vi "Plot Name Write.vi"(4 "error in (no error)":errorcluster, 5 "Value":string, 6 "Container State":T3, 7 "Display State In":T1) -> (0 "error out":errorcluster, 3 "Display State Out":T1)   [LabVIEW 2020, in "XY Plot Matrix.xctl"]
uses:
  <vilib>/Math Plots/2D Math Plots/XY Plot Matrix/XY Plot Matrix XCtrl/XY Plot Matrix.xctl
  <vilib>/_xctls/Container State.ctl
  <vilib>/Math Plots/2D Math Plots/XY Plot Matrix/XY Plot Matrix XCtrl/State.ctl
  <vilib>/Math Plots/2D Math Plots/XY Plot Matrix/XY Plot Matrix/XY Plot Matrix.lvclass
  e:/builds/penguin/labview/branches/2020/dev/dist/vi.lib/Math Plots/2D Math Plots/2D Plot/2D Plot/2D Plot.lvclass
  <vilib>/Math Plots/2D Math Plots/2D Plot/Action String/XYPlotMatrix Ctrl Act Queue.ctl
  <vilib>/Math Plots/2D Math Plots/2D Plot/Action String/XYPlotMatrix Ctrl Act Cluster.ctl
  <vilib>/Math Plots/2D Math Plots/2D Plot/Action String/2DMathPlot State Class.ctl
  <vilib>/Math Plots/2D Math Plots/2D Plot/2D Plot/2D Plot.lvclass
  <vilib>/_xctls/XControlSupport.lvlib
panel:
  # "Replace the Value Control below with a Control of desired type.\nDo not remove this Control or the others from the connector pane.\nDo not change the connector pane pattern.\nThe Value control should always be the third terminal from top on the input side in the connector pane."
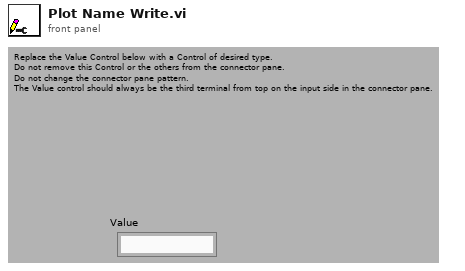
[diagram p1: front panel]
types:
  T1 = typedef "XY Plot Matrix.xctl/State.ctl" = cluster{"XY Plot Matrix.lvclass":refnum<class "XY Plot Matrix.lvclass">, "Control Ref Queue":T2, "Main Frame Color":u32}
  T2 = typedef "XYPlotMatrix Ctrl Act Queue.ctl" = refnum<queue>
  T3 = typedef "XControlSupport.lvlib/Container State.ctl" = cluster{"Indicator?":bool, "Run Mode?":bool, " Refnum":refnum<vi>}
  T4 = typedef "2DMathPlot State Class.ctl" = enum16{"Update All (Undo)", "Update General", "Update Appearance", "Update Format", "Update Scale", "Update Marker", "Update Cursor", "None"}
  T5 = typedef "XY Plot Matrix.lvclass/Plotmatrix Property Array Cluster.ctl" = cluster{"Plotmatrix Property Array":T6, "Active Position":T10}
  T6 = typedef "XY Plot Matrix.lvclass/Plotmatrix Property Array.ctl" = T7[][]
  T7 = typedef "XY Plot Matrix.lvclass/Plotmatrix Property.ctl" = cluster{"Plot Property Array":T8}
  T8 = typedef "2D Plot.lvclass/Plot Property Array.ctl" = T9[]
  T9 = typedef "2D Plot.lvclass/Plot Property.ctl" = cluster{"Bar Plot Style":u8, "DigitalLineStyle":u8, "TransitionLocation":u8, "Transition Type":u8, "Fill To":i16, "Fill/Pt. Color":u32, "Label Style":u8, "Line Style":u8, "Line Width":u8, "Plot Color":u32, "Plot Interpolation":u8, "Plot Name":string, "Point Style":u8, "Visible?":bool, "XScaleIdx":u32, "YScaleIdx":u32}
  T10 = typedef "XY Plot Matrix.lvclass/Active Position.ctl" = cluster{"Row":i32, "Column":i32}
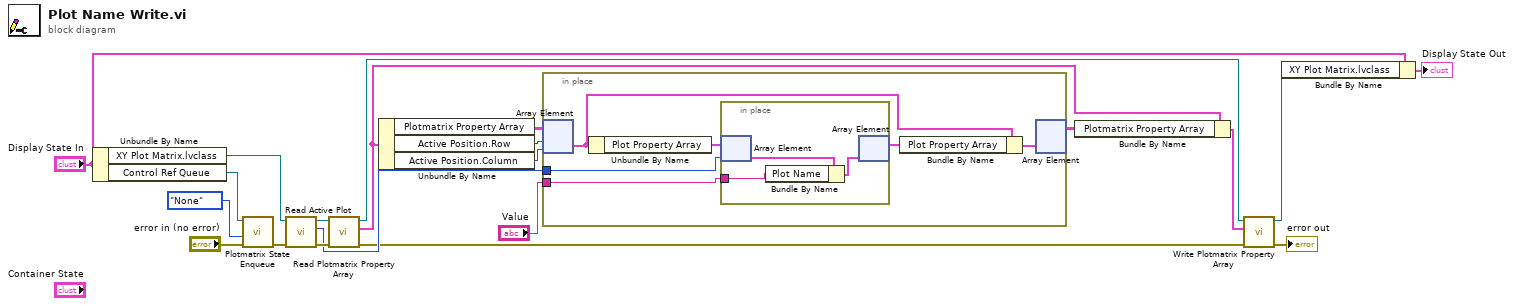
[diagram p0: block diagram]
diagram:
  n1 = Unbundle By Name("Display State In") -> ("XY Plot Matrix.lvclass"=w19:refnum<class "XY Plot Matrix.lvclass">, "Control Ref Queue"=w3:T2)
  n2 = call <vilib>:"Plotmatrix State Enqueue.vi"("error in (no error)"="error in (no error)", "Display State Change Class"=2DMathPlot_State_Class."None", "Control Ref Queue"=w3) -> ("error out"=w1:errorcluster)  [unwired: 8 out]
  n3 = call <vilib>:"Read Active Plot.vi"("error in (no error)"=w1, "2D Plot.lvclass in"=w19) -> ("error out"=w21:errorcluster, "Active Plot"=w15:i32, "2D Plot.lvclass out"=w20:refnum<class "XY Plot Matrix.lvclass">)  [unwired: 7 out]
  n4 = call <vilib>:"Read Plotmatrix Property Array.vi"("error in (no error)"=w21, "2D Plotmatrix.lvclass in"=w20) -> ("error out"=w6:errorcluster, "Plotmatrix Property Array Cluster"=w13:T5, "2D Plotmatrix.lvclass out"=w9:refnum<class "XY Plot Matrix.lvclass">)  [unwired: 7 out]
  n5 = Unbundle By Name(w13) -> ("Plotmatrix Property Array"=w17:T6, "Active Position.Row"=w18:i32, "Active Position.Column"=w16:i32)
  n6 = in-place {
    in-place-border: w15 -> [w26]
    in-place-border: "Value" -> [w25]
    n7 = in-place-array #1(w17, w18, w16) -> (w24:T7)
    n8 = Unbundle By Name(w24) -> ("Plot Property Array"=w27:T8)
    n9 = in-place {
      in-place-border: w25 -> [w29]
      n10 = in-place-array #2(w27, w26) -> (w30:T9)
      n11 = Bundle By Name(cluster=w30, "Plot Name"=w29) -> (w28:T9)
      n12 = in-place-array #2(w28) -> (w23:T8)  [unwired: 1 out]
    }
    n13 = Bundle By Name(cluster=w24, "Plot Property Array"=w23) -> (w22:T7)
    n14 = in-place-array #1(w22) -> (w12:T6)  [unwired: 2 out]
  }
  n15 = Bundle By Name(cluster=w13, "Plotmatrix Property Array"=w12) -> (w11:T5)
  n16 = call <vilib>:"Write Plotmatrix Property Array.vi"("error in (no error)"=w6, "Plotmatrix Property Array Cluster"=w11, "2D Plotmatrix.lvclass in"=w9) -> ("error out"=→"error out":errorcluster, "2D Plotmatrix.lvclass out"=w10:refnum<class "XY Plot Matrix.lvclass">)  [unwired: 7 out]
  n17 = Bundle By Name(cluster="Display State In", "XY Plot Matrix.lvclass"=w10) -> (→"Display State Out":T1)
